vi "SYST_CORR_WIZ.vi"(0 "VISA IN":refnum<visa-resource-name>, 5 "error in":errorcluster, 7 "Type":string(combo)) -> (14 "VISA Out":refnum<visa-resource-name>, 19 "error out":errorcluster)   [LabVIEW 2018, in "PNA-X.lvlib"]
doc: "SYSTem:CORRection:WIZard <char> \n1873\n\n(Write-only) Launches either the Calibration Wizard or the Version 2 Calibration Kit File Manager \ndialog box. \nParameters \n<char> Choose from: \nMAIN - Launches the Calibration Wizard \nCKIT - Launches the Version 2 Calibration Kit File Manager dialog box. \nBoth display on the PNA screen. \nExamples SYST:CORR:WIZ MAIN \nsystem:correction:wizard ckit \nQuery Syntax Not Applicable \nDefault Not Applicable"
uses:
  PNA-X.lvlib
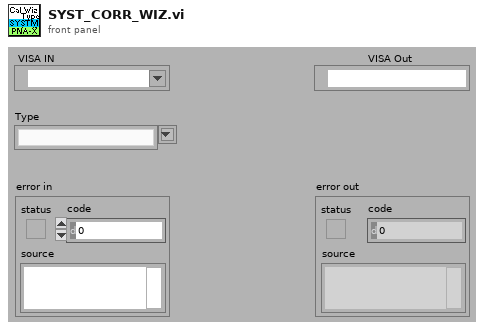
[diagram p1: front panel]
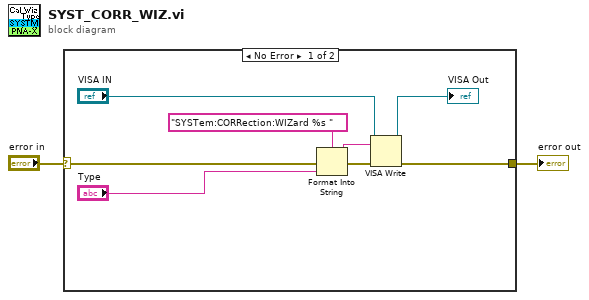
[diagram p0: block diagram]
diagram:
  n1 = case shown="No Error" "error in" {
    selector: "error in" -> [w10 w11]
    tunnel: [w5 w11] -> w1
    frame No Error {
      n2 = Format Into String(format string="SYSTem:CORRection:WIZard %s " ("Cmdline"), error in=w10, "Type") -> (resulting string=w8:string, error out=w9:errorcluster)  [unwired: 1 in]
      n3 = VISA Write(VISA resource name="VISA IN", write buffer=w8, error in (no error)=w9) -> (VISA resource name out=→"VISA Out":refnum<visa-resource-name>, error out=w5:errorcluster)  [unwired: 1 out]
    }
    frame Error {
    }
  }
  "error out" <- w1
